vi "Check for Device Ready.vi"(8 "error in":errorcluster, 11 "VISA resource in":refnum<visa-resource-name>) -> (0 "error out":errorcluster, 2 "device ready?":bool, 3 "VISA resource out":refnum<visa-resource-name>)   [LabVIEW 2018, in "3458A Virtual Digitizer.lvlib" / "3458A Digitizing Low Levels.lvlib"]
doc: "This VI checks device ready flag in the STB. \n\nNote: Reentrant VI so it can be executed in parallel for multiple 3458A sessions."
uses:
  3458A Digitizing Low Levels.lvlib
  3458A Basic Driver/3458A Basic Driver.lvlib
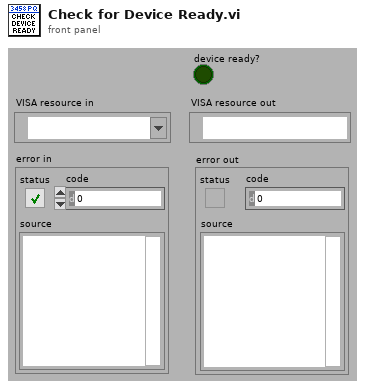
[diagram p1: front panel]
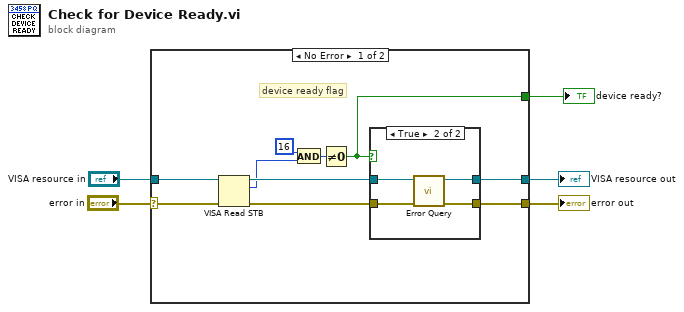
[diagram p0: block diagram]
diagram:
  n1 = case shown="No Error" "error in" {
    selector: "error in" -> [w14 w23]
    tunnel: [w11 w23] -> w3
    tunnel: "VISA resource in" -> [w15 w22]
    tunnel: [w10 w22] -> w2
    tunnel: [w6 _] -> w1
    frame No Error {
      # "device ready flag"
      n2 = VISA Read STB(8:w14, 11:w15) -> (0:w13:errorcluster, 2:w9:u16, 3:w12:refnum<visa-resource-name>)
      n3 = And(x=u16 16, y=w9) -> (x .and. y?=w7:u16)
      n4 = Not Equal To 0?(x=w7) -> (x != 0?=w6:bool)
      n5 = case shown="True" w6 {
        tunnel: w13 -> [w17 w21]
        tunnel: w12 -> [w16 w20]
        tunnel: [w17 w19] -> w11
        tunnel: [w16 w18] -> w10
        frame False {
        }
        frame True {
          n6 = call "Error Query.vi"("error in (no error)"=w21, "VISA resource name"=w20) -> ("error out"=w19:errorcluster, "VISA resource name out"=w18:refnum<visa-resource-name>)  [unwired: 6 in, 2 out]
        }
      }
    }
    frame Error {
    }
  }
  "VISA resource out" <- w2
  "error out" <- w3
  "device ready?" <- w1
